vi "Calculate Loss.vi"   [LabVIEW 2023, in "NI_HFNetworkAnalysis.lvlib"]
doc: "Calculates the mismatch loss of a 2-port network at different frequencies when one of its ports is terminated by the specified termination.\n\nMismatch loss is calculated either using <b>available gain definition</b> or <b>power gain definition</b>.\n\nThe network is defined by 2-port S-parameters <b>(S11,S12,S21,S22)</b> at different frequencies and the termination is described by its reflection factor at those frequencies."
uses:
  NI_HFNetworkAnalysis.lvlib
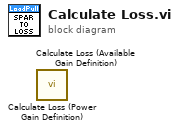
[diagram p0: block diagram]
diagram:
  n1 = call "Calculate Loss (Power Gain Definition).vi"() -> ()  [unwired: 8 in, 2 out]
  n2 = call "Calculate Loss (Available Gain Definition).vi"() -> ()  [unwired: 8 in, 2 out]
